vi "Draft.vi"() -> ()   [LabVIEW 2018]
panel:
  in  "array":bool[](array[boolean])
  out "number":u32
  out "Boolean array 3":bool[](array[boolean])
  in  "Boolean 2":bool
  out "Numeric 2":u8
  out "Boolean array 2":bool[](array[boolean])
  in  "Boolean":bool
  out "Numeric":u8
  out "appended array":bool[][](array[boolean])
  in  "Смещение, до 300_RED":dbl
  out "CmAD3":bool
  out "CmAD2":bool
  out "CmAD1":bool
  out "CmAD0":bool
  in  "Command 2":i16[](array[numeric])=[0, 0, 0, 0, 0, 0, 0, 0, 0, 0, 0, 0, 0, 0, 0, 0, 0, 0, 0, 0, 0, 0, 0, 0, 0, 0, 0, 0, 0, 0, 0, 0, 0, 0, 0, 0, 0, 0, 0, 0, 0, 0, 0, 0, 0]
  out "Boolean array":bool[](array[boolean])
  in  "Data Top":i16[](array[numeric])=[0, 0, 0, 0, 0, 0, 0, 0, 0, 0, 0, 0, 0, 0, 0, 0, 0, 0, 0, 0, 0, 0, 0, 0, 0, 0, 0, 0, 0, 0, 0, 0, 0, 0, 0, 0, 0, 0, 0, 0, 0, 0, 0, 0, 0]
  in  "Command":i16[](array[numeric])=[0, 0, 0, 0, 0, 0, 0, 0, 0, 0, 0, 0, 0, 0, 0, 0, 0, 0, 0, 0, 0, 0, 0, 0, 0, 0, 0, 0, 0, 0, 0, 0, 0, 0, 0, 0, 0, 0, 0, 0, 0, 0, 0, 0, 0]
  in  "Data Bot":i16[](array[numeric])=[0, 0, 0, 0, 0, 0, 0, 0, 0, 0, 0, 0, 0, 0, 0, 0, 0, 0, 0, 0, 0, 0, 0, 0, 0, 0, 0, 0, 0, 0, 0, 0, 0, 0, 0, 0, 0, 0, 0, 0, 0, 0, 0, 0, 0]
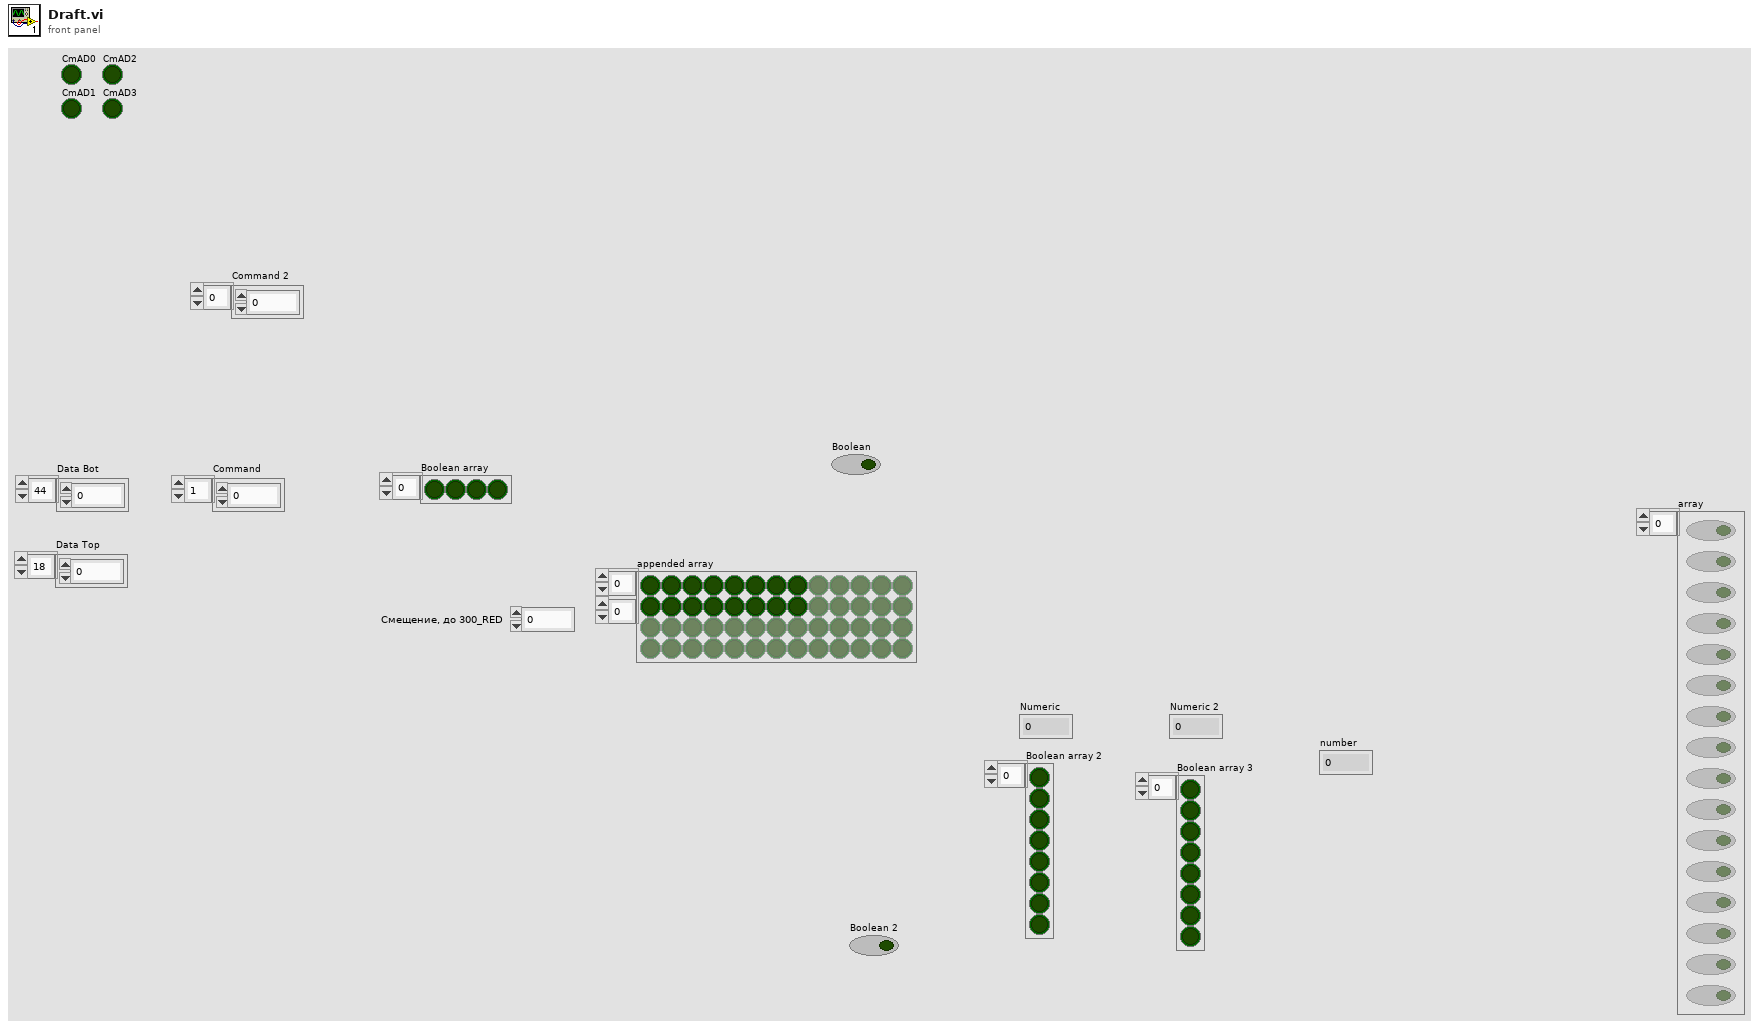
[diagram p1: front panel]
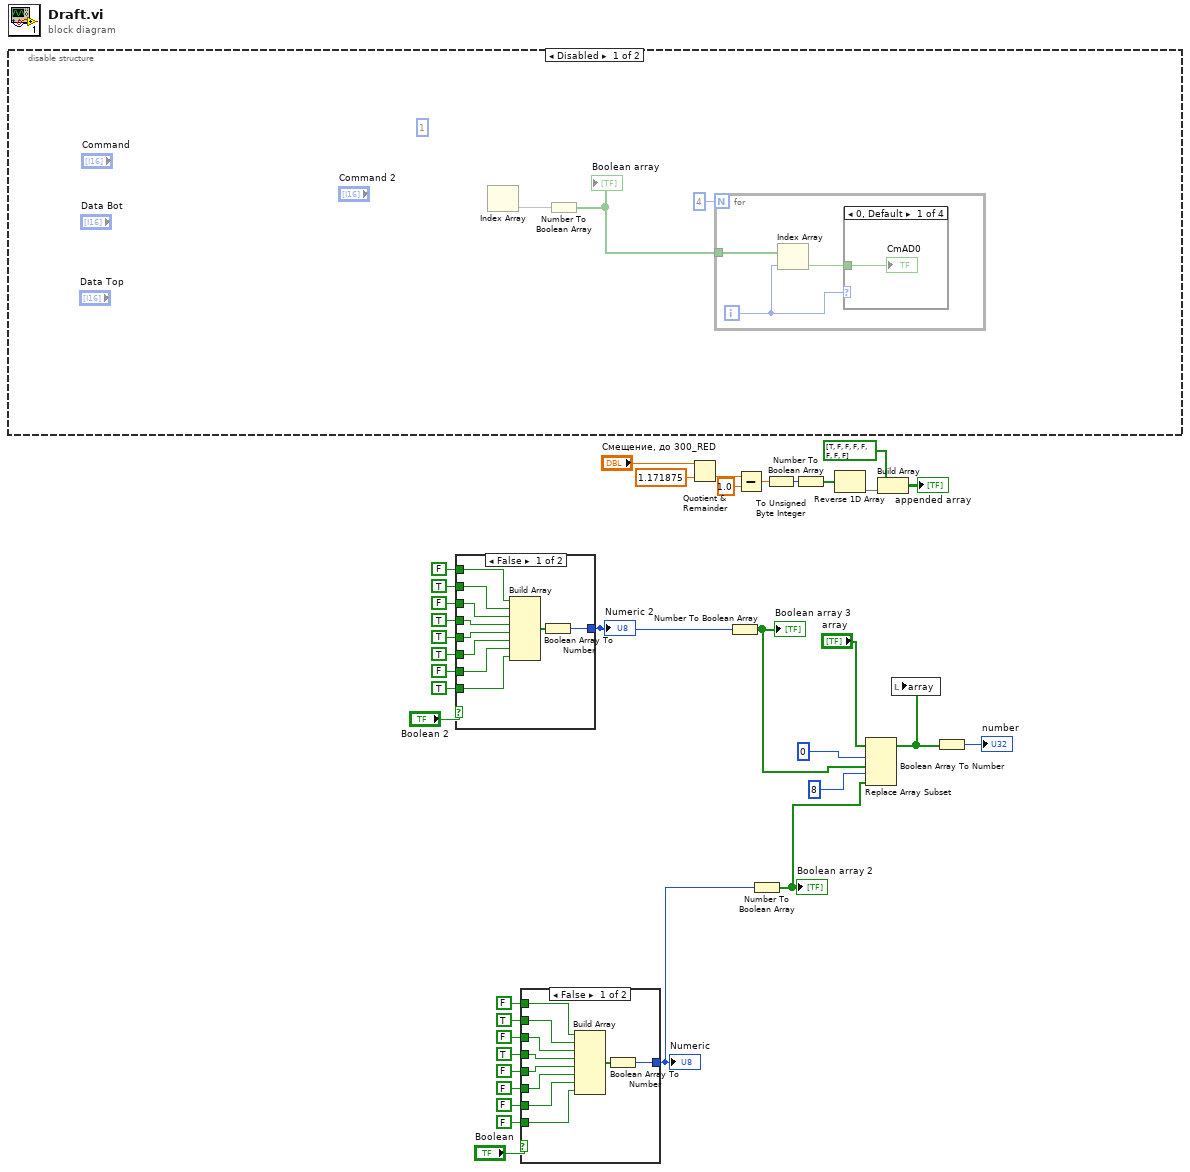
[diagram p0: block diagram]
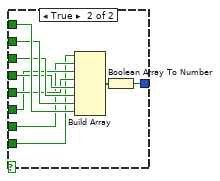
[diagram p2: hidden frame]
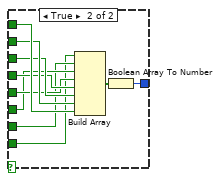
[diagram p3: hidden frame]
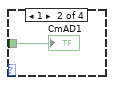
[diagram p4: hidden frame]
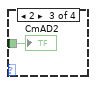
[diagram p5: hidden frame]
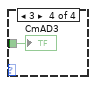
[diagram p6: hidden frame]
diagram:
  n1 = disable-structure shown="Disabled" {
    frame Disabled {
      (unwired) 1
      n2 = Index Array() -> (array=w42:i16[], element=w40, index=w41:i32)
      n3 = Number To Boolean Array(number=w40) -> (Boolean array=w39:bool[])
      "Boolean array" <- w39
      n4 = for {
        N: 4 -> [_]
        tunnel: w39 -> [w45]
        i -> [w44]
        n5 = Index Array(array=w45, index=w44) -> (element=w43:bool)
        n6 = case shown="0, Default" w44 {
          tunnel: w43 -> [w46 w47 w48 w49]
          frame 0, Default {
            "CmAD0" <- w46
          }
          frame 1 {
            "CmAD1" <- w47
          }
          frame 2 {
            "CmAD2" <- w48
          }
          frame 3 {
            "CmAD3" <- w49
          }
        }
      }
    }
    frame Enabled {
    }
  }
  n7 = case shown="False" "Boolean 2" {
    tunnel: FALSE ("IO Module\\DDCA_DIO0_Read") -> [w59 w67]
    tunnel: TRUE ("IO Module\\DDCA_DIO1_Read") -> [w58 w66]
    tunnel: FALSE ("IO Module\\DDCA_DIO2_Read") -> [w57 w65]
    tunnel: TRUE ("IO Module\\DDCA_DIO3_Read") -> [w56 w64]
    tunnel: TRUE ("IO Module\\DDCA_DIO4_Read") -> [w55 w63]
    tunnel: TRUE ("IO Module\\DDCA_DIO5_Read") -> [w54 w62]
    tunnel: FALSE ("IO Module\\DDCA_DIO6_Read") -> [w53 w61]
    tunnel: TRUE ("IO Module\\DDCA_DIO7_Read") -> [w52 w60]
    tunnel: [w50 w68] -> w8
    frame False {
      n8 = Build Array(w59, w58, w57, w56, w55, w54, w53, w52) -> (w51:bool[])
      n9 = Boolean Array To Number(Boolean array=w51) -> (number=w50:u8)
    }
    frame True {
      n10 = Build Array(w60, w61, w62, w63, w64, w65, w66, w67) -> (w69:bool[])
      n11 = Boolean Array To Number(Boolean array=w69) -> (number=w68:u8)
    }
  }
  "Numeric 2" <- w8
  n12 = case shown="False" "Boolean" {
    tunnel: FALSE ("IO Module\\DDCA_DIO0_Read") -> [w79 w87]
    tunnel: TRUE ("IO Module\\DDCA_DIO1_Read") -> [w78 w86]
    tunnel: FALSE ("IO Module\\DDCA_DIO2_Read") -> [w77 w85]
    tunnel: TRUE ("IO Module\\DDCA_DIO3_Read") -> [w76 w84]
    tunnel: FALSE ("IO Module\\DDCA_DIO4_Read") -> [w75 w83]
    tunnel: FALSE ("IO Module\\DDCA_DIO5_Read") -> [w74 w82]
    tunnel: FALSE ("IO Module\\DDCA_DIO6_Read") -> [w73 w81]
    tunnel: FALSE ("IO Module\\DDCA_DIO7_Read") -> [w72 w80]
    tunnel: [w70 w88] -> w18
    frame False {
      n13 = Build Array(w79, w78, w77, w76, w75, w74, w73, w72) -> (w71:bool[])
      n14 = Boolean Array To Number(Boolean array=w71) -> (number=w70:u8)
    }
    frame True {
      n15 = Build Array(w80, w81, w82, w83, w84, w85, w86, w87) -> (w89:bool[])
      n16 = Boolean Array To Number(Boolean array=w89) -> (number=w88:u8)
    }
  }
  "Numeric" <- w18
  n17 = Quotient & Remainder(x="Смещение, до 300_RED", y=1.171875) -> (floor(x/y)=w36:dbl)  [unwired: 1 out]
  n18 = Number To Boolean Array(number=w8) -> (Boolean array=w2:bool[])
  "Boolean array 3" <- w2
  n19 = Subtract(x=w36, y=1.0) -> (x-y=w35:dbl)
  n20 = Number To Boolean Array(number=w18) -> (Boolean array=w1:bool[])
  "Boolean array 2" <- w1
  n21 = To Unsigned Byte Integer(number=w35) -> (unsigned 8bit integer=w34:u8)
  n22 = Number To Boolean Array(number=w34) -> (Boolean array=w33:bool[])
  n23 = Reverse 1D Array(array=w33) -> (reversed array=w32:bool[])
  n24 = Replace Array Subset(array="array", new element #1=w2, index #1=0 ("index"), new element #2=w1, index #2=8 ("index")) -> (w3:bool[])
  n25 = Build Array(bool[] [TRUE, FALSE, FALSE, FALSE, FALSE, FALSE, FALSE, FALSE] ("element"), w32) -> (→"appended array":bool[][])
  n26 = local write "array"(w3) -> ()
  n27 = Boolean Array To Number(Boolean array=w3) -> (number=→"number":u32)
